vi "UI controls access.vi"(8 "error in (no error)":errorcluster, 9 "Sub UI state":string, 10 "Main UI State":string, 11 "Controls and Indicators\nReferences":T1) -> (0 "error out":errorcluster)   [LabVIEW 2019, in "ZenGage v3.0 UI.lvclass"]
uses:
  ZenGage v3.0 UI.lvclass
  Type Definitions/Controls and Indicators/Select a part (combobox).ctl
  Type Definitions/Controls and Indicators/EDL control references.ctl
  Type Definitions/Controls and Indicators/Diagnostics control referencs.ctl
  Type Definitions/Controls and Indicators/Inspection control references.ctl
  Type Definitions/Controls and Indicators/General_Control references.ctl
  Type Definitions/Controls and Indicators/Controls and Indicators Cluster.ctl
  Type Definitions/General/Master sample references.ctl
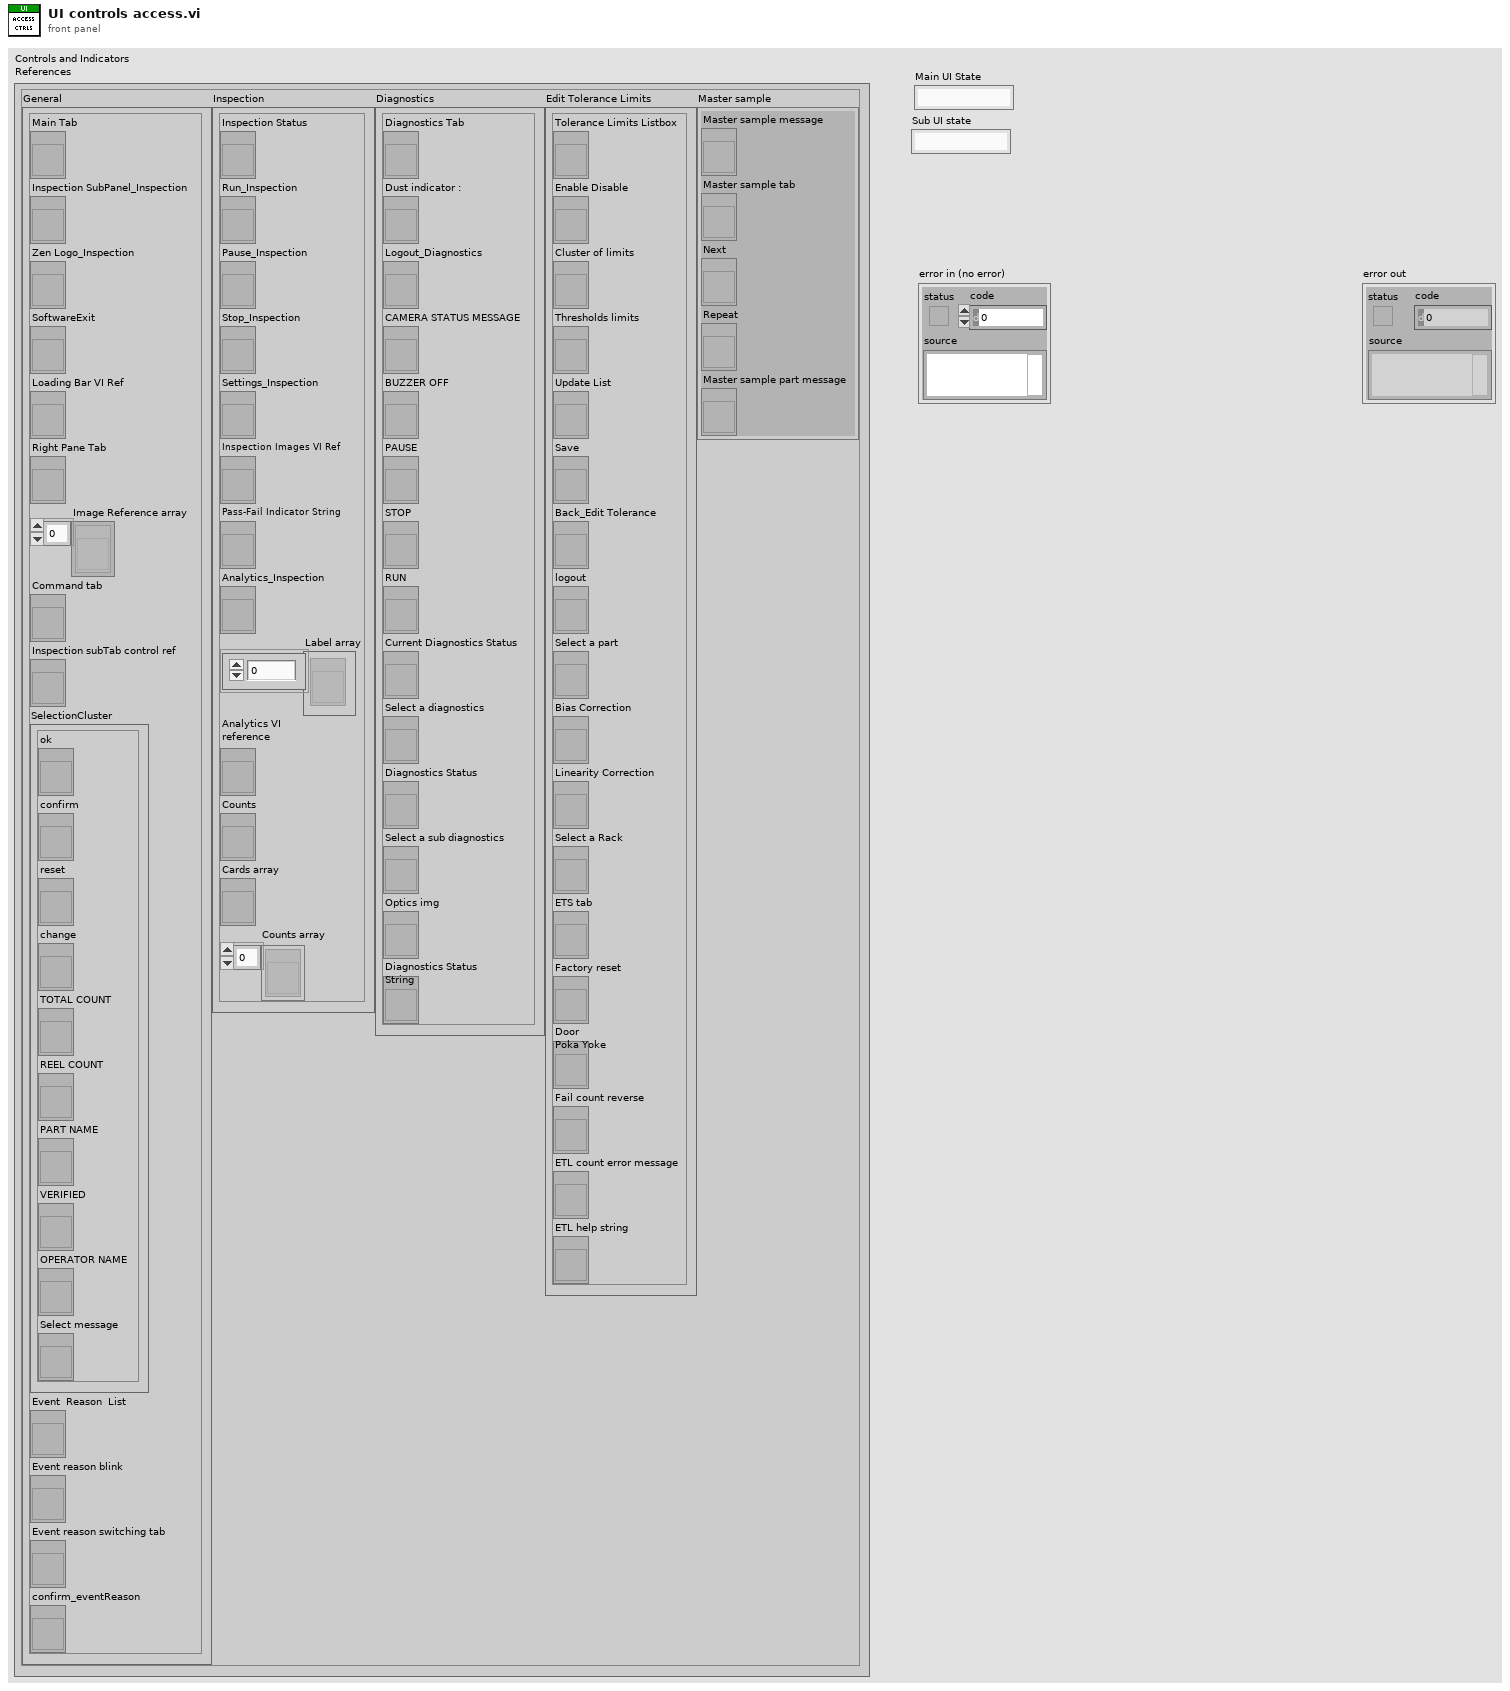
[diagram p1: front panel]
types:
  T1 = typedef "ZenGage v3.0 UI.lvclass/Controls and Indicators Cluster.ctl" = cluster{"General":T2, "Inspection":T3, "Diagnostics":T4, "Edit Tolerance Limits":T5, "Master sample":T6}
  T2 = typedef "ZenGage v3.0 UI.lvclass/General_Control references.ctl" = cluster{"Main Tab":refnum<vi>, "Inspection SubPanel_Inspection":refnum<vi>, "Zen Logo_Inspection":refnum<vi>, "SoftwareExit":refnum<vi>, "Loading Bar VI Ref":refnum<vi>, "Right Pane Tab":refnum<vi>, "Image Reference array":refnum<vi>[], "Command tab":refnum<vi>, "Inspection subTab control ref":refnum<vi>, "SelectionCluster":cluster{"ok":refnum<vi>, "confirm":refnum<vi>, "reset":refnum<vi>, "change":refnum<vi>, "TOTAL COUNT":refnum<vi>, "REEL COUNT":refnum<vi>, "PART NAME":refnum<vi>, "VERIFIED":refnum<vi>, "OPERATOR NAME":refnum<vi>, "Select message":refnum<vi>}, "Event  Reason  List":refnum<vi>, "Event reason blink":refnum<vi>, "Event reason switching tab":refnum<vi>, "confirm_eventReason":refnum<vi>}
  T3 = typedef "ZenGage v3.0 UI.lvclass/Inspection control references.ctl" = cluster{"Inspection Status":refnum<vi>, "Run_Inspection":refnum<vi>, "Pause_Inspection":refnum<vi>, "Stop_Inspection":refnum<vi>, "Settings_Inspection":refnum<vi>, "Inspection Images VI Ref":refnum<vi>, "Pass-Fail Indicator String":refnum<vi>, "Analytics_Inspection":refnum<vi>, "Label array":refnum<vi>[], "Analytics VI\nreference":refnum<vi>, "Counts":refnum<vi>, "Cards array":refnum<vi>, "Counts array":refnum<vi>[]}
  T4 = typedef "ZenGage v3.0 UI.lvclass/Diagnostics control referencs.ctl" = cluster{"Diagnostics Tab":refnum<vi>, "Dust indicator :":refnum<vi>, "Logout_Diagnostics":refnum<vi>, "CAMERA STATUS MESSAGE":refnum<vi>, "BUZZER OFF":refnum<vi>, "PAUSE":refnum<vi>, "STOP":refnum<vi>, "RUN":refnum<vi>, "Current Diagnostics Status":refnum<vi>, "Select a diagnostics":refnum<vi>, "Diagnostics Status":refnum<vi>, "Select a sub diagnostics":refnum<vi>, "Optics img":refnum<vi>, "Diagnostics Status\nString":refnum<vi>}
  T5 = typedef "ZenGage v3.0 UI.lvclass/EDL control references.ctl" = cluster{"Tolerance Limits Listbox":refnum<vi>, "Enable Disable":refnum<vi>, "Cluster of limits":refnum<vi>, "Thresholds limits":refnum<vi>, "Update List":refnum<vi>, "Save":refnum<vi>, "Back_Edit Tolerance":refnum<vi>, "logout":refnum<vi>, "Select a part":refnum<vi>, "Bias Correction":refnum<vi>, "Linearity Correction":refnum<vi>, "Select a Rack":refnum<vi>, "ETS tab":refnum<vi>, "Factory reset":refnum<vi>, "Door\nPoka Yoke":refnum<vi>, "Fail count reverse":refnum<vi>, "ETL count error message":refnum<vi>, "ETL help string":refnum<vi>}
  T6 = typedef "Master sample references.ctl" = cluster{"Master sample message":refnum<vi>, "Master sample tab":refnum<vi>, "Next":refnum<vi>, "Repeat":refnum<vi>, "Master sample part message":refnum<vi>}
  T7 = enum32{"Edit Tolerance Limits1", "Inspection", "Master sample", "Diagnostics"}
  T8 = enum8{"Enabled", "Disabled", "Disabled and Grayed Out"}
  T9 = enum32{"Analytics", "Blank", "Diagnostics", "Run", "Edit Tolerance Settings"}
  T10 = enum32{"Inspection", "Diagnostics", "Edit Tolerance Settings"}
  T11 = enum32{"Arduino Motor", "Sensor trigger", "Hardware Button", "Camera Optics"}
  T12 = cluster{"Measruement Name":string, "Measruement pass?":bool, "LSL":string, "USL 2":string, "Measurement value":dbl}[]
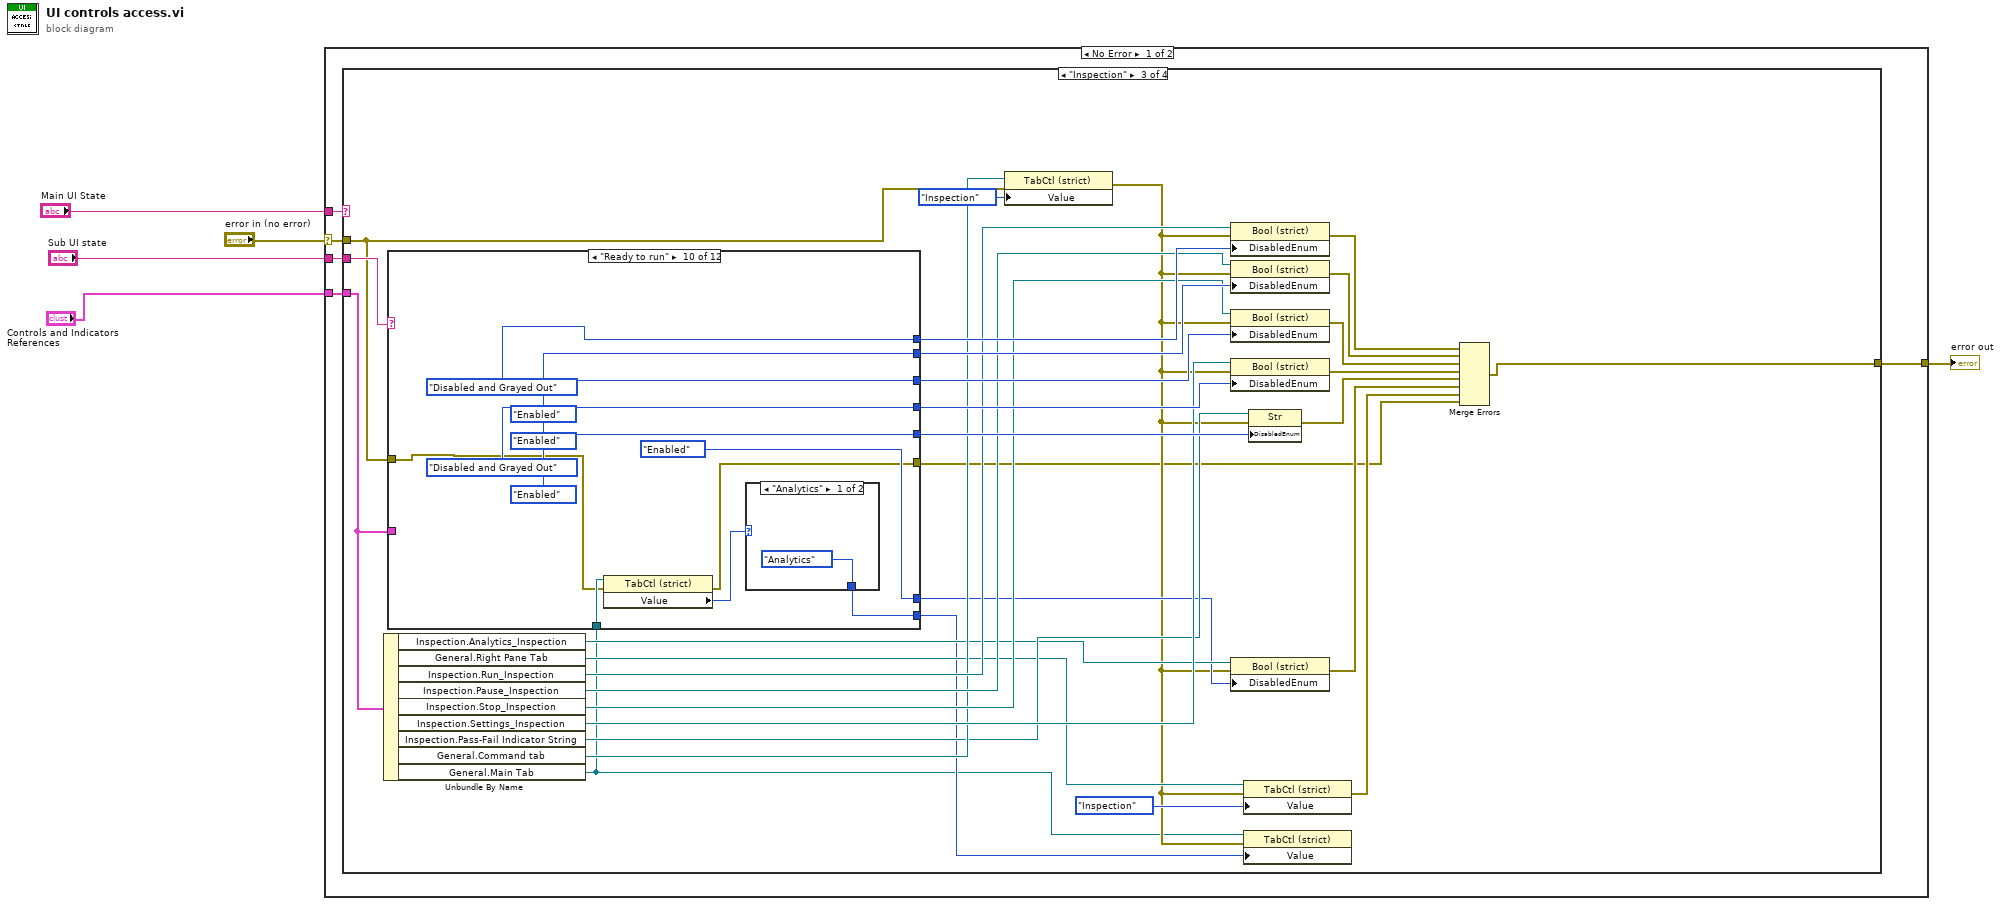
[diagram p0: block diagram]
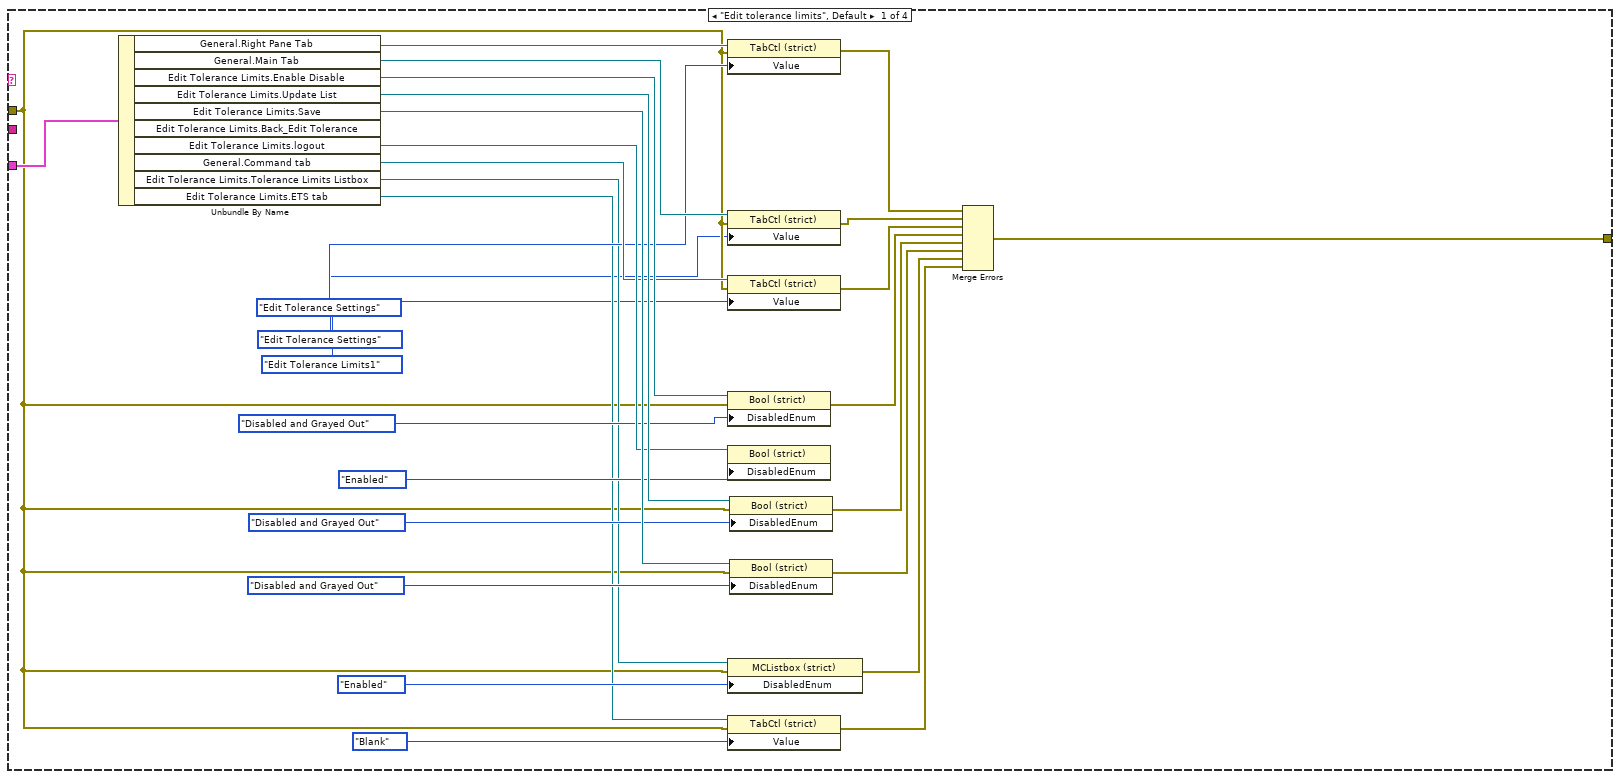
[diagram p2: hidden frame]
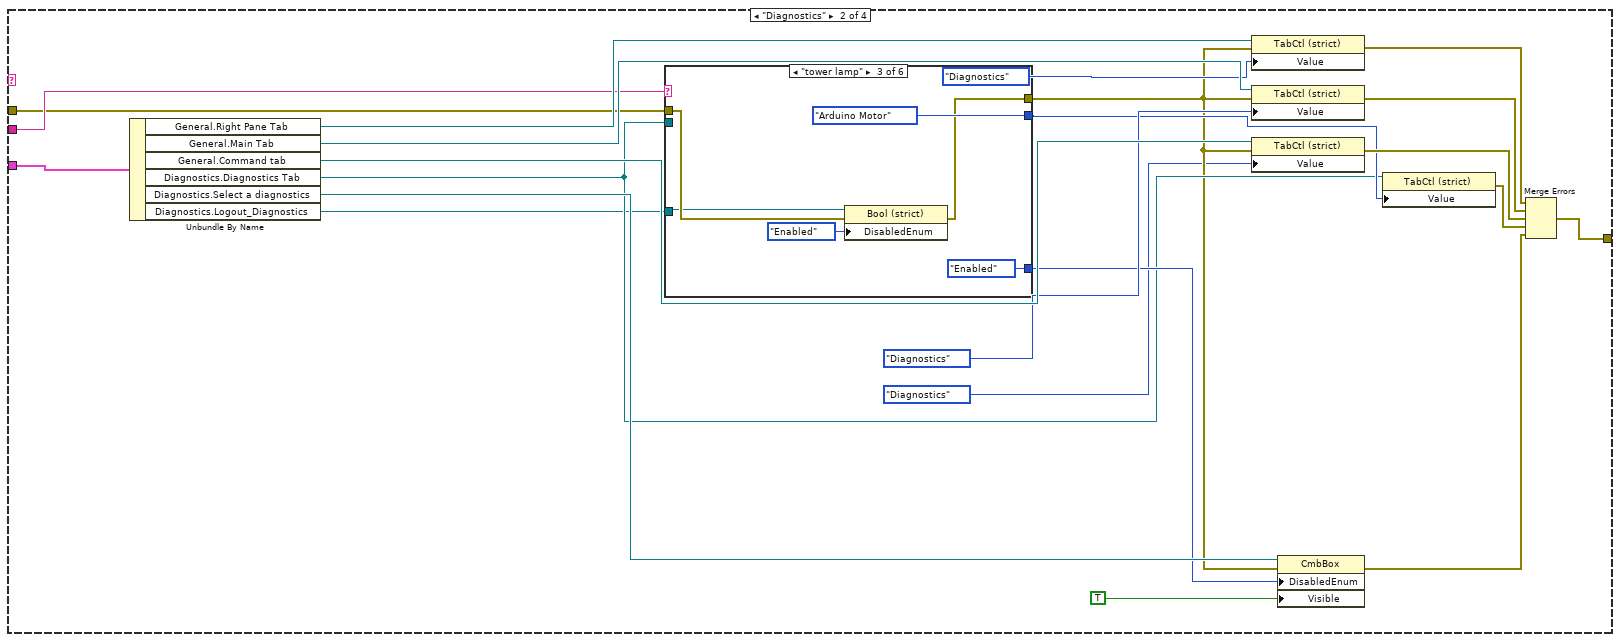
[diagram p3: hidden frame]
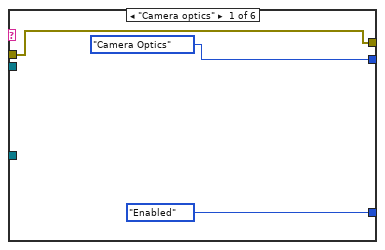
[diagram p4: hidden frame]
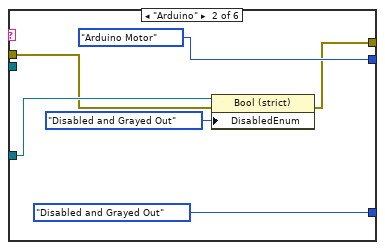
[diagram p5: hidden frame]
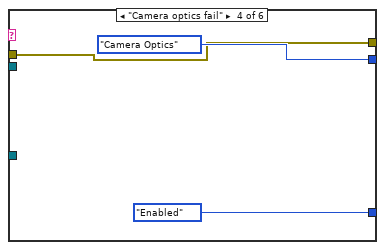
[diagram p6: hidden frame]
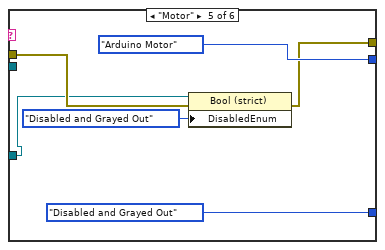
[diagram p7: hidden frame]
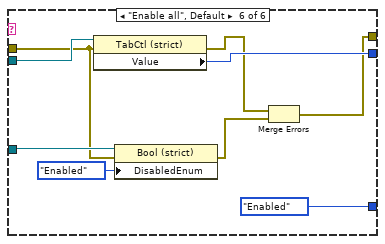
[diagram p8: hidden frame]
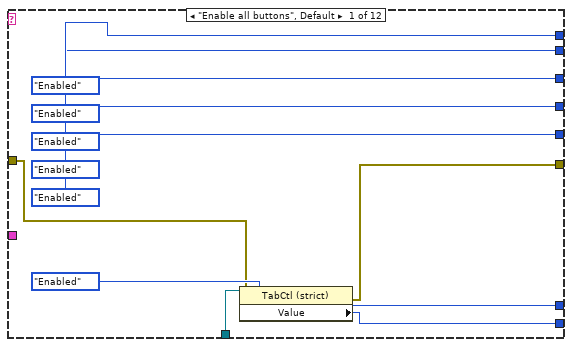
[diagram p9: hidden frame]
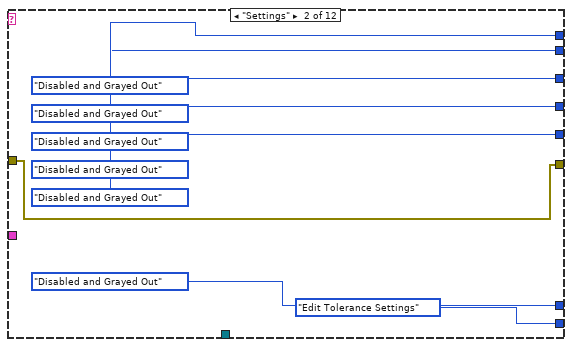
[diagram p10: hidden frame]
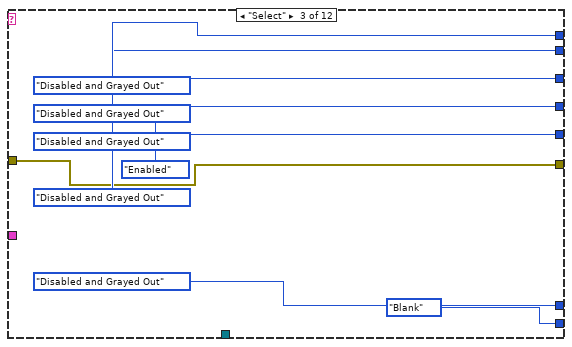
[diagram p11: hidden frame]
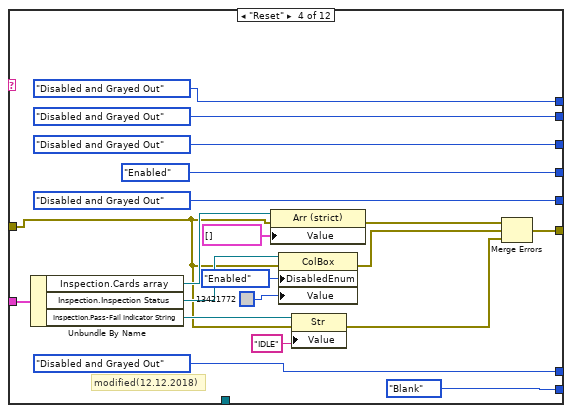
[diagram p12: hidden frame]
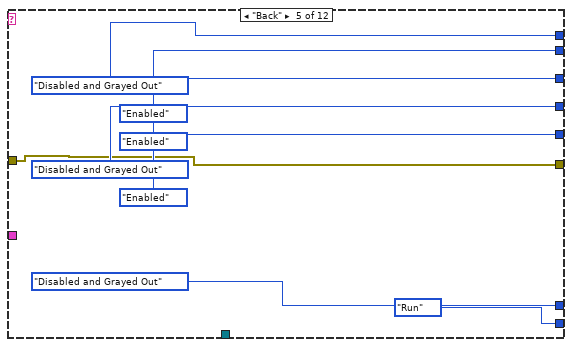
[diagram p13: hidden frame]
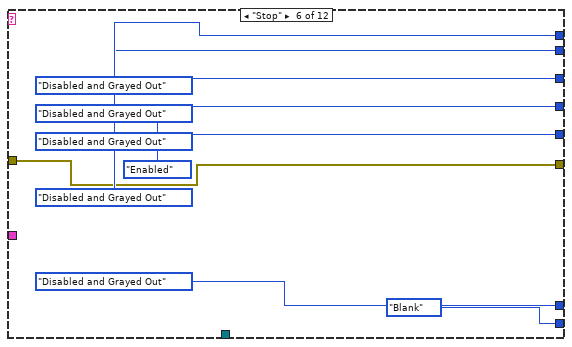
[diagram p14: hidden frame]
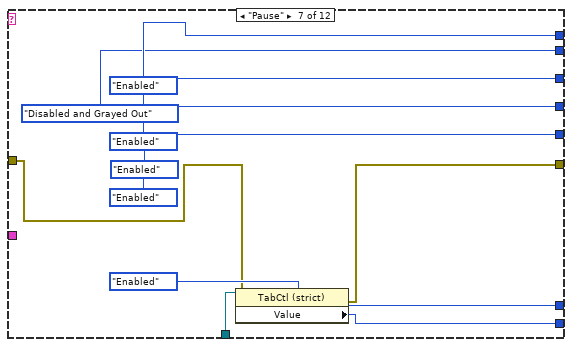
[diagram p15: hidden frame]
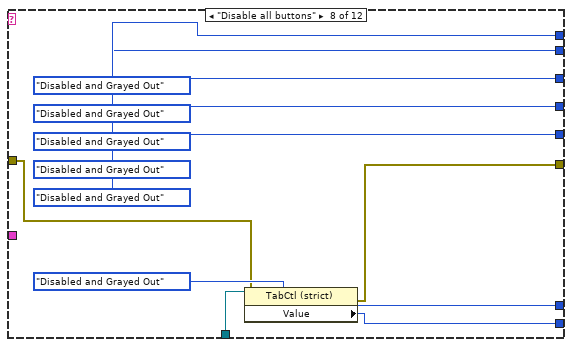
[diagram p16: hidden frame]
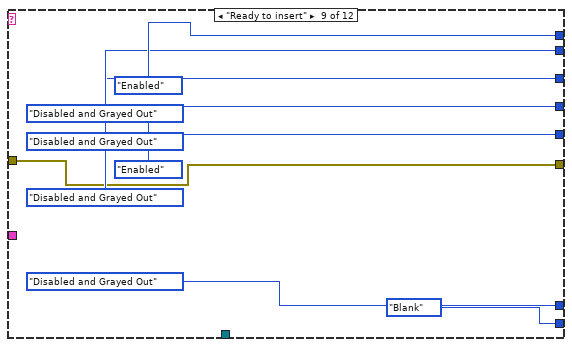
[diagram p17: hidden frame]
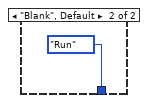
[diagram p18: hidden frame]
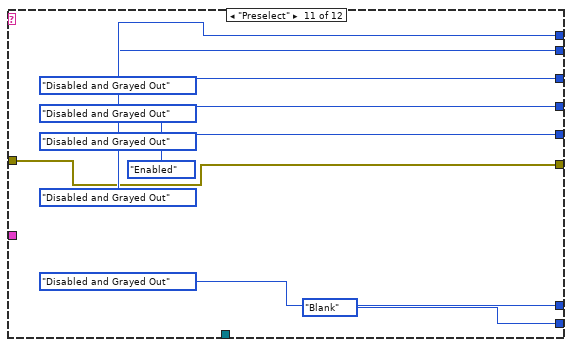
[diagram p19: hidden frame]
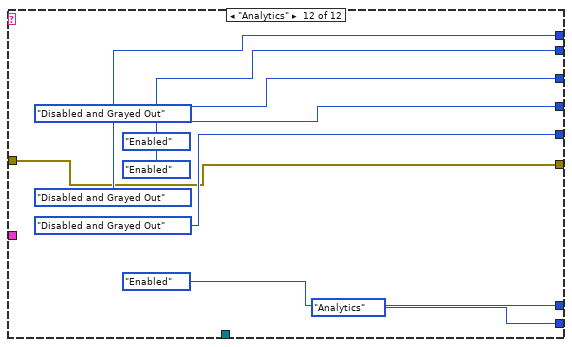
[diagram p20: hidden frame]
diagram:
  n1 = case shown="No Error" "error in (no error)" {
    selector: "error in (no error)" -> [w9 w300]
    tunnel: "Controls and Indicators\nReferences" -> [w10 _]
    tunnel: [w8 w300] -> w4
    tunnel: "Main UI State" -> [w7 _]
    tunnel: "Sub UI state" -> [w6 _]
    frame No Error {
      n2 = case shown="\"Inspection\"" w7 {
        tunnel: w10 -> [w39 w61 w96 w248]
        tunnel: w9 -> [w13 w45 w98 w247]
        tunnel: [w32 w55 w109 w246] -> w8
        tunnel: w6 -> [_ w50 w106 w245]
        frame "Edit tolerance limits", Default {
          n3 = Unbundle By Name(w39) -> ("General.Right Pane Tab"=w31:refnum<vi>, "General.Main Tab"=w34:refnum<vi>, "Edit Tolerance Limits.Enable Disable"=w35:refnum<vi>, "Edit Tolerance Limits.Update List"=w38:refnum<vi>, "Edit Tolerance Limits.Save"=w37:refnum<vi>, "Edit Tolerance Limits.logout"=w36:refnum<vi>, "General.Command tab"=w33:refnum<vi>, "Edit Tolerance Limits.Tolerance Limits Listbox"=w20:refnum<vi>, "Edit Tolerance Limits.ETS tab"=w18:refnum<vi>)  [unwired: 1 out]
          n4 = property class="TabCtl (strict)"(reference=w31, error in=w13, "Value"=T10."Edit Tolerance Settings") -> (error out=w14:errorcluster)  [unwired: 1 out]
          n5 = property class="TabCtl (strict)"(reference=w34, error in=w13, "Value"=T9."Edit Tolerance Settings") -> (error out=w15:errorcluster)  [unwired: 1 out]
          n6 = property class="TabCtl (strict)"(reference=w33, error in=w13, "Value"=T7."Edit Tolerance Limits1") -> (error out=w26:errorcluster)  [unwired: 1 out]
          n7 = property class="Bool (strict)"(reference=w35, error in=w13, "DisabledEnum"=T8."Disabled and Grayed Out" ("Disabled")) -> (error out=w25:errorcluster)  [unwired: 1 out]
          n8 = property class="Bool (strict)"(reference=w36, "DisabledEnum"=T8."Enabled" ("Disabled")) -> ()  [unwired: 1 in, 2 out]
          n9 = property class="MCListbox (strict)"(reference=w20, error in=w13, "DisabledEnum"=T8."Enabled" ("Disabled")) -> (error out=w21:errorcluster)  [unwired: 1 out]
          n10 = property class="TabCtl (strict)"(reference=w18, error in=w13, "Value"=enum32{"Display", "Blank"}."Blank") -> (error out=w16:errorcluster)  [unwired: 1 out]
          n11 = property class="Bool (strict)"(reference=w38, error in=w13, "DisabledEnum"=T8."Disabled and Grayed Out" ("Disabled")) -> (error out=w24:errorcluster)  [unwired: 1 out]
          n12 = property class="Bool (strict)"(reference=w37, error in=w13, "DisabledEnum"=T8."Disabled and Grayed Out" ("Disabled")) -> (error out=w23:errorcluster)  [unwired: 1 out]
          n13 = Merge Errors(w14, w15, w26, w25, w24, w23, w21, w16) -> (w32:errorcluster)
        }
        frame "Diagnostics" {
          n14 = Unbundle By Name(w61) -> ("General.Right Pane Tab"=w53:refnum<vi>, "General.Main Tab"=w60:refnum<vi>, "General.Command tab"=w59:refnum<vi>, "Diagnostics.Diagnostics Tab"=w46:refnum<vi>, "Diagnostics.Select a diagnostics"=w49:refnum<vi>, "Diagnostics.Logout_Diagnostics"=w41:refnum<vi>)
          n15 = case shown="\"tower lamp\"" w50 {
            tunnel: [T11."Camera Optics" ("Value") T11."Arduino Motor" ("Value") T11."Arduino Motor" ("Value") T11."Camera Optics" ("Value") T11."Arduino Motor" ("Value") w92] -> w51
            tunnel: [T8."Enabled" ("Disabled") T8."Disabled and Grayed Out" ("Disabled") T8."Enabled" ("Disabled") T8."Enabled" ("Disabled") T8."Disabled and Grayed Out" ("Disabled") T8."Enabled" ("Disabled")] -> w48
            tunnel: w46 -> [_ _ _ _ _ w93]
            tunnel: w45 -> [w62 w66 w74 w77 w82 w89]
            tunnel: [w62 w65 w73 w77 w81 w86] -> w42
            tunnel: w41 -> [_ w67 w71 _ w80 w91]
            frame "Camera optics" {
            }
            frame "Arduino" {
              n16 = property class="Bool (strict)"(reference=w67, error in=w66, "DisabledEnum"=T8."Disabled and Grayed Out" ("Disabled")) -> (error out=w65:errorcluster)  [unwired: 1 out]
            }
            frame "tower lamp" {
              n17 = property class="Bool (strict)"(reference=w71, error in=w74, "DisabledEnum"=T8."Enabled" ("Disabled")) -> (error out=w73:errorcluster)  [unwired: 1 out]
            }
            frame "Camera optics fail" {
            }
            frame "Motor" {
              n18 = property class="Bool (strict)"(reference=w80, error in=w82, "DisabledEnum"=T8."Disabled and Grayed Out" ("Disabled")) -> (error out=w81:errorcluster)  [unwired: 1 out]
            }
            frame "Enable all", Default {
              n19 = property class="TabCtl (strict)"(reference=w93, error in=w89) -> (error out=w87:errorcluster, "Value"=w92:T11)  [unwired: 1 out]
              n20 = property class="Bool (strict)"(reference=w91, error in=w89, "DisabledEnum"=T8."Enabled" ("Disabled")) -> (error out=w88:errorcluster)  [unwired: 1 out]
              n21 = Merge Errors(w87, w88) -> (w86:errorcluster)
            }
          }
          n22 = property class="TabCtl (strict)"(reference=w53, error in=w42, "Value"=T10."Diagnostics") -> (error out=w43:errorcluster)  [unwired: 1 out]
          n23 = property class="TabCtl (strict)"(reference=w60, error in=w42, "Value"=T9."Diagnostics") -> (error out=w58:errorcluster)  [unwired: 1 out]
          n24 = property class="TabCtl (strict)"(reference=w59, error in=w42, "Value"=T7."Diagnostics") -> (error out=w57:errorcluster)  [unwired: 1 out]
          n25 = property class="CmbBox"(reference=w49, error in=w42, "DisabledEnum"=w48, "Visible"=TRUE) -> (error out=w47:errorcluster)  [unwired: 1 out]
          n26 = property class="TabCtl (strict)"(reference=w46, "Value"=w51) -> (error out=w56:errorcluster)  [unwired: 1 in, 1 out]
          n27 = Merge Errors(w43, w58, w57, w56, w47) -> (w55:errorcluster)
        }
        frame "Inspection" {
          n28 = Unbundle By Name(w96) -> ("Inspection.Analytics_Inspection"=w105:refnum<vi>, "General.Right Pane Tab"=w107:refnum<vi>, "Inspection.Run_Inspection"=w120:refnum<vi>, "Inspection.Pause_Inspection"=w119:refnum<vi>, "Inspection.Stop_Inspection"=w118:refnum<vi>, "Inspection.Settings_Inspection"=w117:refnum<vi>, "Inspection.Pass-Fail Indicator String"=w115:refnum<vi>, "General.Command tab"=w116:refnum<vi>, "General.Main Tab"=w99:refnum<vi>)
          n29 = case shown="\"Ready to run\"" w106 {
            tunnel: [T8."Enabled" ("Disabled") T8."Disabled and Grayed Out" ("Disabled") T8."Disabled and Grayed Out" ("Disabled") T8."Disabled and Grayed Out" ("Disabled") T8."Disabled and Grayed Out" ("Disabled") T8."Disabled and Grayed Out" ("Disabled") T8."Enabled" ("Disabled") T8."Disabled and Grayed Out" ("Disabled") T8."Enabled" ("Disabled") T8."Disabled and Grayed Out" ("Disabled") T8."Disabled and Grayed Out" ("Disabled") T8."Disabled and Grayed Out" ("Disabled")] -> w125
            tunnel: [T8."Enabled" ("Disabled") T8."Disabled and Grayed Out" ("Disabled") T8."Disabled and Grayed Out" ("Disabled") T8."Disabled and Grayed Out" ("Disabled") T8."Enabled" ("Disabled") T8."Disabled and Grayed Out" ("Disabled") T8."Disabled and Grayed Out" ("Disabled") T8."Disabled and Grayed Out" ("Disabled") T8."Disabled and Grayed Out" ("Disabled") T8."Enabled" ("Disabled") T8."Disabled and Grayed Out" ("Disabled") T8."Enabled" ("Disabled")] -> w124
            tunnel: [T8."Enabled" ("Disabled") T8."Disabled and Grayed Out" ("Disabled") T8."Disabled and Grayed Out" ("Disabled") T8."Disabled and Grayed Out" ("Disabled") T8."Enabled" ("Disabled") T8."Disabled and Grayed Out" ("Disabled") T8."Enabled" ("Disabled") T8."Disabled and Grayed Out" ("Disabled") T8."Disabled and Grayed Out" ("Disabled") T8."Enabled" ("Disabled") T8."Disabled and Grayed Out" ("Disabled") T8."Enabled" ("Disabled")] -> w123
            tunnel: [T8."Enabled" ("Disabled") T8."Disabled and Grayed Out" ("Disabled") T8."Enabled" ("Disabled") T8."Enabled" ("Disabled") T8."Disabled and Grayed Out" ("Disabled") T8."Enabled" ("Disabled") T8."Enabled" ("Disabled") T8."Disabled and Grayed Out" ("Disabled") T8."Enabled" ("Disabled") T8."Disabled and Grayed Out" ("Disabled") T8."Enabled" ("Disabled") T8."Disabled and Grayed Out" ("Disabled")] -> w122
            tunnel: [T8."Enabled" ("Disabled") T8."Disabled and Grayed Out" ("Disabled") T8."Disabled and Grayed Out" ("Disabled") T8."Disabled and Grayed Out" ("Disabled") T8."Enabled" ("Disabled") T8."Disabled and Grayed Out" ("Disabled") T8."Enabled" ("Disabled") T8."Disabled and Grayed Out" ("Disabled") T8."Disabled and Grayed Out" ("Disabled") T8."Enabled" ("Disabled") T8."Disabled and Grayed Out" ("Disabled") T8."Disabled and Grayed Out" ("Disabled")] -> w121
            tunnel: [T8."Enabled" ("Disabled") T8."Disabled and Grayed Out" ("Disabled") T8."Disabled and Grayed Out" ("Disabled") T8."Disabled and Grayed Out" ("Disabled") T8."Disabled and Grayed Out" ("Disabled") T8."Disabled and Grayed Out" ("Disabled") T8."Enabled" ("Disabled") T8."Disabled and Grayed Out" ("Disabled") T8."Disabled and Grayed Out" ("Disabled") T8."Enabled" ("Disabled") T8."Disabled and Grayed Out" ("Disabled") T8."Enabled" ("Disabled")] -> w104
            tunnel: [w127 T9."Edit Tolerance Settings" ("Value") T9."Blank" ("Value") T9."Blank" ("Value") T9."Run" ("Value") T9."Blank" ("Value") w189 w199 T9."Blank" ("Value") w216 T9."Blank" ("Value") T9."Analytics" ("Value")] -> w100
            tunnel: w99 -> [w129 _ _ _ _ _ w191 w201 _ w220 _ _]
            tunnel: w98 -> [w128 w136 w144 w158 w172 w180 w190 w200 w208 w219 w229 w237]
            tunnel: w96 -> [_ _ _ w164 _ _ _ _ _ _ _ _]
            tunnel: [w126 w136 w144 w154 w172 w180 w188 w198 w208 w218 w229 w237] -> w95
            frame "Enable all buttons", Default {
              n30 = property class="TabCtl (strict)"(reference=w129, error in=w128) -> (error out=w126:errorcluster, "Value"=w127:T9)  [unwired: 1 out]
            }
            frame "Settings" {
            }
            frame "Select" {
            }
            frame "Reset" {
              # "modified(12.12.2018)"
              n31 = Unbundle By Name(w164) -> ("Inspection.Cards array"=w163:refnum<vi>, "Inspection.Inspection Status"=w162:refnum<vi>, "Inspection.Pass-Fail Indicator String"=w161:refnum<vi>)
              n32 = property class="Arr (strict)"(reference=w163, error in=w158, "Value"=T12 []) -> (error out=w157:errorcluster)  [unwired: 1 out]
              n33 = property class="ColBox"(reference=w162, error in=w158, "DisabledEnum"=T8."Enabled" ("Disabled"), "Value"=u32 13421772) -> (error out=w156:errorcluster)  [unwired: 1 out]
              n34 = property class="Str"(reference=w161, error in=w158, "Value"="IDLE") -> (error out=w155:errorcluster)  [unwired: 1 out]
              n35 = Merge Errors(w157, w156, w155) -> (w154:errorcluster)
            }
            frame "Back" {
            }
            frame "Stop" {
            }
            frame "Pause" {
              n36 = property class="TabCtl (strict)"(reference=w191, error in=w190) -> (error out=w188:errorcluster, "Value"=w189:T9)  [unwired: 1 out]
            }
            frame "Disable all buttons" {
              n37 = property class="TabCtl (strict)"(reference=w201, error in=w200) -> (error out=w198:errorcluster, "Value"=w199:T9)  [unwired: 1 out]
            }
            frame "Ready to insert" {
            }
            frame "Ready to run" {
              n38 = property class="TabCtl (strict)"(reference=w220, error in=w219) -> (error out=w218:errorcluster, "Value"=w217:T9)  [unwired: 1 out]
              n39 = case shown="\"Analytics\"" w217 {
                tunnel: [T9."Analytics" ("Value") T9."Run" ("Value")] -> w216
                frame "Analytics" {
                }
                frame "Blank", Default {
                }
              }
            }
            frame "Preselect" {
            }
            frame "Analytics" {
            }
          }
          n40 = property class="TabCtl (strict)"(reference=w116, error in=w98, "Value"=T7."Inspection") -> (error out=w101:errorcluster)  [unwired: 1 out]
          n41 = property class="Bool (strict)"(reference=w120, error in=w101, "DisabledEnum"=w125) -> (error out=w114:errorcluster)  [unwired: 1 out]
          n42 = property class="Bool (strict)"(reference=w119, error in=w101, "DisabledEnum"=w124) -> (error out=w113:errorcluster)  [unwired: 1 out]
          n43 = property class="Bool (strict)"(reference=w118, error in=w101, "DisabledEnum"=w123) -> (error out=w112:errorcluster)  [unwired: 1 out]
          n44 = property class="Bool (strict)"(reference=w117, error in=w101, "DisabledEnum"=w122) -> (error out=w111:errorcluster)  [unwired: 1 out]
          n45 = property class="Bool (strict)"(reference=w105, error in=w101, "DisabledEnum"=w104) -> (error out=w103:errorcluster)  [unwired: 1 out]
          n46 = property class="TabCtl (strict)"(reference=w107, error in=w101, "Value"=T10."Inspection") -> (error out=w102:errorcluster)  [unwired: 1 out]
          n47 = property class="TabCtl (strict)"(reference=w99, error in=w101, "Value"=w100) -> ()  [unwired: 2 out]
          n48 = property class="Str"(reference=w115, error in=w101, "DisabledEnum"=w121) -> (error out=w110:errorcluster)  [unwired: 1 out]
          n49 = Merge Errors(w114, w113, w112, w111, w110, w103, w102, w95) -> (w109:errorcluster)
        }
        frame "Master sample" {
          n50 = case shown="\"Initialize master sample\"" w245 {
            tunnel: w248 -> [_ w258 w264 w284 w293]
            tunnel: w247 -> [w249 w253 w260 w283 w292]
            tunnel: [w249 w250 w263 w282 w291] -> w246
            frame "False", Default {
            }
            frame "Move to next sample" {
              n51 = Unbundle By Name(w258) -> ("Master sample.Next"=w257:refnum<vi>, "Master sample.Repeat"=w255:refnum<vi>)
              n52 = property class="Bool (strict)"(reference=w257, error in=w253, "DisabledEnum"=T8."Enabled" ("Disabled")) -> (error out=w251:errorcluster)  [unwired: 1 out]
              n53 = property class="Bool (strict)"(reference=w255, error in=w253, "DisabledEnum"=T8."Disabled and Grayed Out" ("Disabled")) -> (error out=w252:errorcluster)  [unwired: 1 out]
              n54 = Merge Errors(w251, w252) -> (w250:errorcluster)
            }
            frame "Initialize master sample" {
              w278 = T8."Disabled and Grayed Out" ("Disabled")
              n55 = Unbundle By Name(w264) -> ("General.Right Pane Tab"=w262:refnum<vi>, "General.Main Tab"=w268:refnum<vi>, "General.Command tab"=w270:refnum<vi>, "Master sample.Master sample tab"=w281:refnum<vi>, "Master sample.Next"=w280:refnum<vi>, "Master sample.Repeat"=w279:refnum<vi>, "Master sample.Master sample part message"=w273:refnum<vi>)
              n56 = property class="TabCtl (strict)"(reference=w262, error in=w260, "Value"=T10."Inspection") -> (error out=w259:errorcluster)  [unwired: 1 out]
              n57 = property class="TabCtl (strict)"(reference=w268, error in=w260, "Value"=T9."Run") -> (error out=w266:errorcluster)  [unwired: 1 out]
              n58 = property class="TabCtl (strict)"(reference=w270, error in=w260, "Value"=T7."Master sample") -> (error out=w269:errorcluster)  [unwired: 1 out]
              n59 = property class="TabCtl (strict)"(reference=w281, error in=w260, "Value"=enum32{"Master sample", "Inspection"}."Master sample") -> (error out=w277:errorcluster)  [unwired: 1 out]
              n60 = property class="Bool (strict)"(reference=w280, error in=w260, "DisabledEnum"=w278) -> (error out=w276:errorcluster)  [unwired: 1 out]
              n61 = property class="Bool (strict)"(reference=w279, error in=w260, "DisabledEnum"=w278) -> (error out=w275:errorcluster)  [unwired: 1 out]
              n62 = property class="Str"(reference=w273, error in=w260, "Value"="") -> (error out=w271:errorcluster)  [unwired: 1 out]
              n63 = Merge Errors(w259, w266, w269, w277, w276, w275, w271) -> (w263:errorcluster)
            }
            frame "Master sample validation pass" {
              n64 = Unbundle By Name(w284) -> ("Master sample.Next"=w290:refnum<vi>, "Master sample.Repeat"=w289:refnum<vi>)
              n65 = property class="Bool (strict)"(reference=w290, error in=w283, "DisabledEnum"=T8."Enabled" ("Disabled")) -> (error out=w286:errorcluster)  [unwired: 1 out]
              n66 = property class="Bool (strict)"(reference=w289, error in=w283, "DisabledEnum"=T8."Enabled" ("Disabled")) -> (error out=w285:errorcluster)  [unwired: 1 out]
              n67 = Merge Errors(w286, w285) -> (w282:errorcluster)
            }
            frame "Master sample validation fail" {
              n68 = Unbundle By Name(w293) -> ("Master sample.Next"=w297:refnum<vi>, "Master sample.Repeat"=w296:refnum<vi>)
              n69 = property class="Bool (strict)"(reference=w297, error in=w292, "DisabledEnum"=T8."Disabled and Grayed Out" ("Disabled")) -> (error out=w299:errorcluster)  [unwired: 1 out]
              n70 = property class="Bool (strict)"(reference=w296, error in=w292, "DisabledEnum"=T8."Enabled" ("Disabled")) -> (error out=w298:errorcluster)  [unwired: 1 out]
              n71 = Merge Errors(w299, w298) -> (w291:errorcluster)
            }
          }
        }
      }
    }
    frame Error {
    }
  }
  "error out" <- w4
